vi "Analyze.vi"(8 "error in (no error)":errorcluster, 10 "Image in":T1, 11 "Analyze Distanz in":refnum<class "Analyze BeamDeviation.lvclass">) -> (0 "error out":errorcluster, 1 "Result":refnum<class "Analyze Results Base.lvclass">, 2 "Image out":T1, 3 "Analyze Distanz out":refnum<class "Analyze BeamDeviation.lvclass">)   [LabVIEW 2014, in "Analyze.lvlib" / "Analyze BeamDeviation.lvclass"]
uses:
  Analyze BeamDeviation.lvclass
  <vilib>/vision/Image Controls.llb/IMAQ Image.ctl
  Results and Overlays/Results Base/Analyze Results Base.lvclass
  Results and Overlays/Results Beam Deviation/Analyze Results Beam Deviation.lvclass
  Analyze Parameter/Analyze Parameter Target Point/Target Point.lvclass
  Analyze Parameter/Analyze Parameter Target Point/Target Point.lvclass/Target Point.ctl
  Results and Overlays/Results Base/Analyze Results Base.lvclass/Analyze Results Base.ctl
  Results and Overlays/Results Beam Deviation/Analyze Results Beam Deviation.lvclass/Analyze Results Beam Deviation.ctl
  Results and Overlays/Results Base/Write Position.vi
  Results and Overlays/Results Beam Deviation/Write Delta.vi
  Analyze BaseClass/Analyze BaseClass/Analyze BaseClass.lvclass
  <vilib>/vision/NI_Vision_Development_Module.lvlib
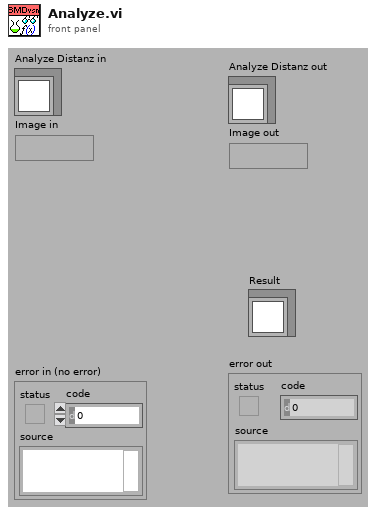
[diagram p1: front panel]
types:
  T1 = typedef "IMAQ Image.ctl" = refnum<image>
  T2 = typedef "ROI Descriptor" = cluster{"Global Rectangle":i32[], "Contours":cluster{"ID":enum32{"External", "Internal"}, "Type":u32, "Coordinates":i32[]}[]}
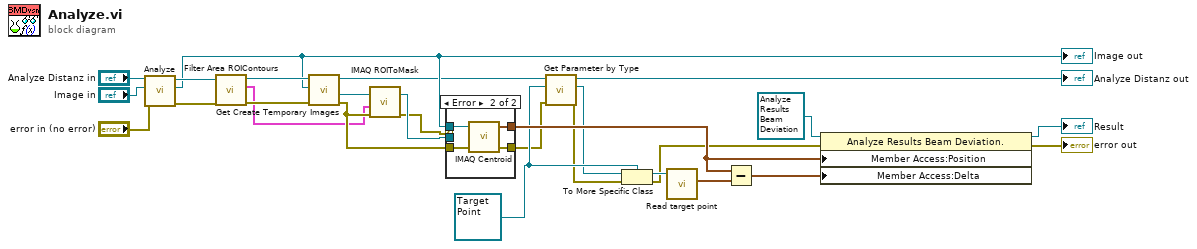
[diagram p0: block diagram]
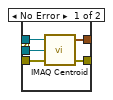
[diagram p2: hidden frame]
diagram:
  w5 = refnum<class "Target Point.lvclass"> refnum ("Target Point.lvclass")
  n1 = call-parent "Analyze.vi"("error in (no error)"="error in (no error)", "Image in"="Image in", "Analyze BaseClass in"="Analyze Distanz in") -> ("error out"=w17:errorcluster, "Image out"=w15:T1, "Analyze BaseClass out"=w18:refnum<class "Analyze BeamDeviation.lvclass">)  [unwired: 5 in, 1 out]
  "Image out" <- w15
  n2 = call-dynamic "Filter Area ROIContours.vi"("error in (no error)"=w17, "Analyze BaseClass in"=w18) -> ("error out"=w26:errorcluster, "ROI of Area type"=w21:T2, "Analyze BaseClass out"=w27:refnum<class "Analyze BeamDeviation.lvclass">)  [unwired: 7 in]
  n3 = call-dynamic "Get Create Temporary Images.vi"("error in (no error)"=w26, "Image in"=w15, "Analyze BaseClass in"=w27) -> ("error out"=w23:errorcluster, "image mask"=w25:T1, "Analyze BaseClass out"=w12:refnum<class "Analyze BeamDeviation.lvclass">)  [unwired: 4 in, 2 out]
  n4 = call "IMAQ ROIToMask"("error in (no error)"=w23, "ROI Descriptor"=w21, "Image"=w25) -> ("error out"=w22:errorcluster, "Image Out"=w24:T1)  [unwired: 3 in, 1 out]
  n5 = case shown="Error" w22 {
    tunnel: w15 -> [w32 w36]
    tunnel: w24 -> [w31 _]
    tunnel: [w30 w35] -> w3
    tunnel: [w29 w34] -> w8
    tunnel: w23 -> [w28 w33]
    frame No Error {
      n6 = call "IMAQ Centroid"("error in (no error)"=w28, "Image Mask"=w31, "Image"=w32) -> ("error out"=w30:errorcluster, "Centroid"=w29:cluster{"X Centroid":sgl, "Y Centroid":sgl})  [unwired: 1 in]
    }
    frame Error {
      n7 = call "IMAQ Centroid"("error in (no error)"=w33, "Image"=w36) -> ("error out"=w35:errorcluster, "Centroid"=w34:cluster{"X Centroid":sgl, "Y Centroid":sgl})  [unwired: 2 in]
    }
  }
  n8 = call "Get Parameter by Type.vi"("error in (no error)"=w3, "Parameter Type"=w5, "Analyze BaseClass in"=w12) -> ("error out"=w2:errorcluster, "Parameter"=w4:refnum<class "Analyze Parameter Base.lvclass">, "Analyze BaseClass out"=→"Analyze Distanz out":refnum<class "Analyze BeamDeviation.lvclass">)  [unwired: 5 in, 1 out]
  n9 = To More Specific Class(target class=w5, reference=w4, error in=w2) -> (specific class reference=w7:refnum<class "Target Point.lvclass">, error out=w1:errorcluster)
  n10 = call "Read target point.vi"("Target Point in"=w7) -> ("target point"=w14:cluster{"x":i16, "y":i16})  [unwired: 8 in, 2 out]
  n11 = Subtract(x=w8, y=w14) -> (x-y=w9:cluster{sgl, sgl})
  n12 = property class="Analyze Results Beam Deviation."(reference=refnum<class "Analyze Results Beam Deviation.lvclass"> refnum ("Analyze Results Beam Deviation.lvclass"), error in=w1, "Member Access:Position"=w8, "Member Access:Delta"=w9) -> (reference out=→"Result":refnum<class "Analyze Results Beam Deviation.lvclass">, error out=→"error out":errorcluster)
